vi "conversor de tramas.vi"() -> ()   [LabVIEW 2021]
panel:
  out "array":string[](array[string])
  out "text":string
  in  "file (use dialog)":path
  out "Array 3":u8[](array[numeric])
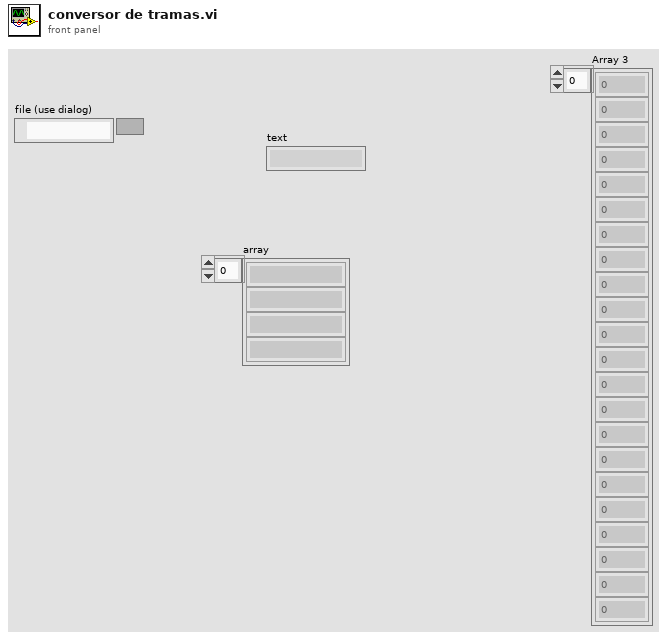
[diagram p1: front panel]
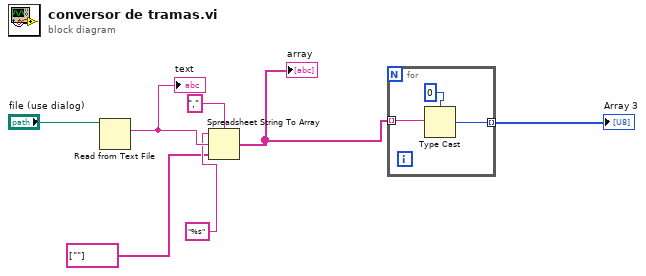
[diagram p0: block diagram]
diagram:
  n1 = Read from Text File(file (use dialog)="file (use dialog)") -> (text=w5:string)  [unwired: 3 in, 3 out]
  "text" <- w5
  n2 = Spreadsheet String To Array(delimiter (Tab)=",", format string="%s", spreadsheet string=w5, array type (2D Dbl)=string[] [""] ("Array 5")) -> (array=w1:string[])
  "array" <- w1
  n3 = for {
    tunnel: [w9] -> w7 mode=indexing
    tunnel: w1 -> [w8] mode=indexing
    n4 = Type Cast(type=u8 0 ("unsigned 8bit integer"), x=w8) -> (*(type *) &x=w9:u8)
  }
  "Array 3" <- w7
